vi "SubVI_file_all.vi"(8 "err in":errorcluster caption="에러 입력(에러 없음)") -> (0 "err out":errorcluster caption="에러 출력")   [LabVIEW 2016]
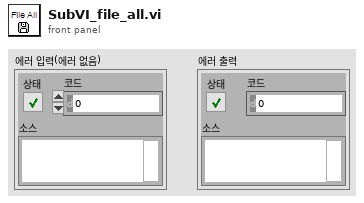
[diagram p1: front panel]
types:
  T1 = enum16{"create", "write_data", "write_event", "read_data", "read_event", "close"}
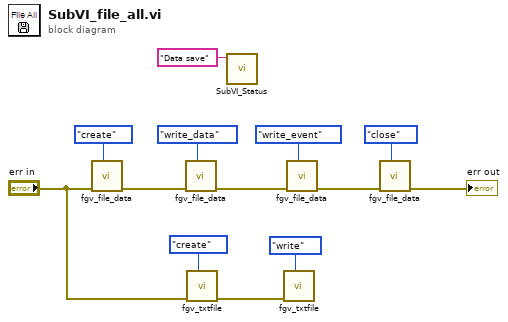
[diagram p0: block diagram]
diagram:
  n1 = call "fgv_file_data.vi"("cmd_file"=T1."create", "err in"="err in") -> ("error out"=w11:errorcluster)  [unwired: 6 in, 3 out]
  n2 = call "fgv_file_data.vi"("cmd_file"=T1."write_data", "err in"=w11) -> ("error out"=w7:errorcluster)  [unwired: 6 in, 3 out]
  n3 = call "fgv_txtfile.vi"("cmd"=enum16{"write", "create"}."create", "err in"="err in") -> ("error out"=w5:errorcluster)  [unwired: 9 in]
  n4 = call "SubVI_Status.vi"("info_str"="Data save") -> ()  [unwired: 10 in, 1 out]
  n5 = call "fgv_txtfile.vi"("cmd"=enum16{"write", "create"}."write", "err in"=w5) -> ()  [unwired: 9 in, 1 out]
  n6 = call "fgv_file_data.vi"("cmd_file"=T1."write_event", "err in"=w7) -> ("error out"=w12:errorcluster)  [unwired: 6 in, 3 out]
  n7 = call "fgv_file_data.vi"("cmd_file"=T1."close", "err in"=w12) -> ("error out"=→"err out":errorcluster)  [unwired: 6 in, 3 out]
